vi "XML Template File.vi"(11 "CD Template":refnum<class "NIVS_PPL_Inline HW Interface.lvclass">) -> (2 "XML Template File":path)   [LabVIEW 2020, in "NIVS_PPL_Inline HW Interface.lvclass"]
uses:
  NIVS_PPL_Inline HW Interface.lvclass
  NIVS_Consolidated_CDW_MetaDataObj/XML File.ctl
  NIVS_Consolidated_CDW_MetaDataObj/XML File.vi
  NIVS_Consolidated_CDW_MetaDataObj/NIVS_Consolidated_CDW_MetaDataObj.lvclass
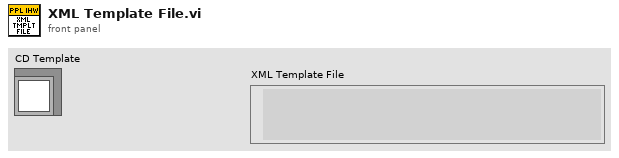
[diagram p1: front panel]
types:
  T1 = typedef "NIVS_Consolidated_CDW_MetaDataObj.lvclass/XML File.ctl" = enum16{"XMLTemplateFilePathAndName", "XMLTimingAndSyncFileName", "XMLCustomDeviceFileName", "XMLTemplateFilePathAndName (Inline-Async)", "XMLPPLTemplateFilePathAndName (Inline-Async)", "XMLPPLTemplateFilePathAndName (Inline)"}
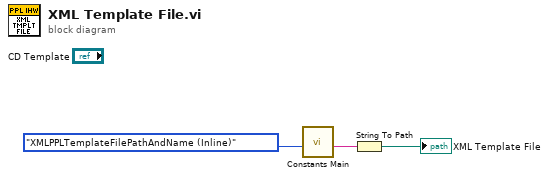
[diagram p0: block diagram]
diagram:
  n1 = call-poly "Constants Main.vi"("Action"=XML_File."XMLPPLTemplateFilePathAndName (Inline)") -> ("Output"=w3:string)  [unwired: 10 in]
  n2 = String To Path(string=w3) -> (path=→"XML Template File":path)
